vi "Do.vi"(6 "Input":variant, 8 "error in":errorcluster, 9 "Self Enqueuer":refnum<class "Message Enqueuer.lvclass">, 10 "Series Enqueuer":refnum<class "Message Enqueuer.lvclass">, 11 "Sample Tacho Fan in":refnum<class "Sample Tacho Fan.lvclass">) -> (0 "error out":errorcluster, 3 "Sample Tacho Fan out":refnum<class "Sample Tacho Fan.lvclass">)   [LabVIEW 2023, in "Sample Tacho Fan.lvclass"]
uses:
  Sample Tacho Fan.lvclass
  D:/git/HAL/HAL GOOP4/Task/Task Base/Task Base.lvclass
  <vilib>/ActorFramework/Message Enqueuer/Message Enqueuer.lvclass
  Task/ITask Actor/ITask Actor Messages/Do Msg/Do Msg.lvclass
  C:/Program Files/National Instruments/LabVIEW 2023/vi.lib/ActorFramework/Message/Message.lvclass
  Task/Task Base/Task Base.lvclass/Task Base.ctl
  Series/ISeries Actor/ISeries Actor Messages/Point Data Updated Msg/Point Data Updated Msg.lvclass/Point Data Updated Msg.ctl
  <vilib>/ActorFramework/Message Enqueuer/Message Enqueuer.lvclass/Message Enqueuer.ctl
  <vilib>/ActorFramework/Message Enqueuer/Enqueue.vi
  Series/ISeries Actor/ISeries Actor Messages/Point Data Updated Msg/Point Data Updated Msg.lvclass
  <vilib>/Utility/LVClass/Get LV Class Name.vi
  <resource>/AFDebug/Generate Trace for Message.vi
  <vilib>/ActorFramework/Message Priority Queue/Priority Enqueue.vi
  Task/Task Base/Task Base.lvclass
  Measure and Stimulus Subsystems/Measure and Stimulus Subsystems.lvclass
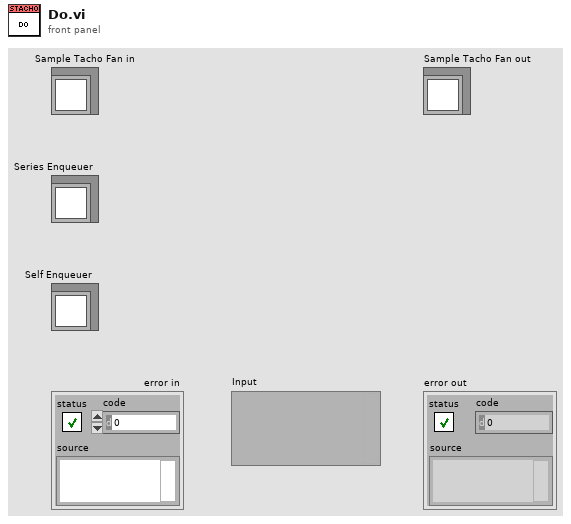
[diagram p1: front panel]
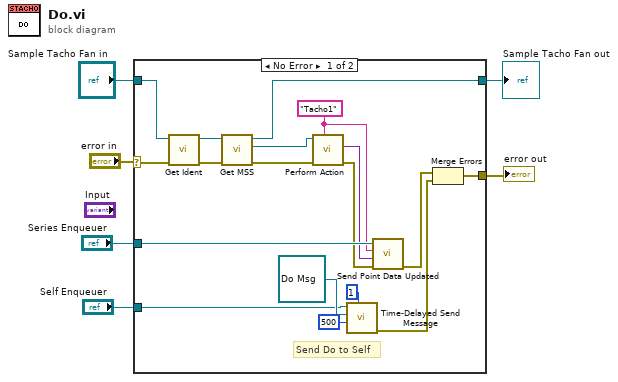
[diagram p0: block diagram]
diagram:
  n1 = case shown="No Error" "error in" {
    selector: "error in" -> [w23 w26]
    tunnel: [w24 w26] -> w6
    tunnel: [w22 w25] -> w5
    tunnel: "Sample Tacho Fan in" -> [w19 w25]
    tunnel: "Series Enqueuer" -> [w21 _]
    tunnel: "Self Enqueuer" -> [w13 _]
    frame No Error {
      w10 = "Tacho1" ("Target Identifier")
      # "Send Do to Self"
      n2 = call "Get Ident.vi"("error in (no error)"=w23, "Task Base in"=w19) -> ("error out"=w20:errorcluster, "Task Base out"=w18:refnum<class "Sample Tacho Fan.lvclass">)  [unwired: 7 in, 1 out]
      n3 = call "Get MSS.vi"("error in (no error)"=w20, "Task Base in"=w18) -> ("error out"=w12:errorcluster, "MSS"=w11:refnum<class "Measure and Stimulus Subsystems.lvclass">, "Task Base out"=w22:refnum<class "Sample Tacho Fan.lvclass">)  [unwired: 7 in]
      n4 = call "Perform Action.vi"("Point Ident"=w10, "error in"=w12, "MSS in"=w11) -> ("error out"=w7:errorcluster, "Output"=w17:variant)  [unwired: 6 in, 1 out]
      n5 = call <vilib>:"Time-Delayed Send Message.vi"("# Copies (0 = infinite repeat)"=u32 1, "Milliseconds To Wait"=500, "Message"=refnum<class "Do Msg.lvclass"> refnum ("HAL GOOP4.lvlib:ITask Actor.lvlib:Do Msg.lvclass"), "Message Enqueuer"=w13) -> ("error out"=w9:errorcluster)  [unwired: 6 in, 1 out]
      n6 = call "Send Point Data Updated.vi"("error in (no error)"=w7, "Data"=w17, "Point Ident"=w10, "Message Enqueuer"=w21) -> ("error out"=w8:errorcluster)  [unwired: 6 in, 1 out]
      n7 = Merge Errors(w8, w9) -> (w24:errorcluster)
    }
    frame Error {
    }
  }
  "error out" <- w6
  "Sample Tacho Fan out" <- w5
